vi "PQnparams.vi"(8 "error in (no error)":errorcluster, 10 "res":u64) -> (0 "error out":errorcluster, 1 "PQnparams":u64, 2 "res_out":u64)   [LabVIEW 2019, in "libpqlv64.lvlib"]
uses:
  libpqlv64.lvlib
  libpq.dll
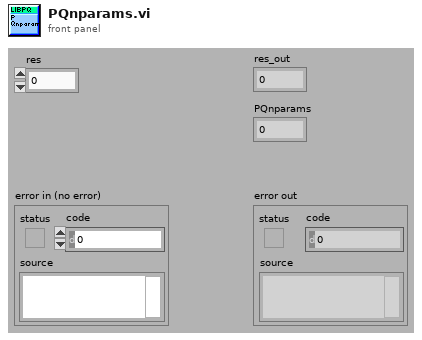
[diagram p1: front panel]
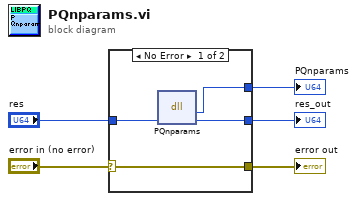
[diagram p0: block diagram]
diagram:
  n1 = case shown="No Error" "error in (no error)" {
    selector: "error in (no error)" -> [w9 w11]
    tunnel: [w9 w11] -> w4
    tunnel: [w8 _] -> w3
    tunnel: "res" -> [w7 w10]
    tunnel: [w6 w10] -> w1
    frame No Error {
      n2 = dll-call lib="libpq.*" fn="PQnparams"("res"=w7) -> ("PQnparams"=w8:u64, "res"=w6:u64)  [unwired: 3 in, 2 out]
    }
    frame Error {
    }
  }
  "PQnparams" <- w3
  "error out" <- w4
  "res_out" <- w1
